vi "Post logout actions.vi"(6 "Cluster out":T2, 7 "Label.Text":string, 8 "error in (no error)":errorcluster, 9 "Caller Enqueuer":refnum<class "Message Enqueuer.lvclass">, 10 "Self Enqueuer":refnum<class "Message Enqueuer.lvclass">, 11 "ControlsIndicators":T3) -> (0 "error out":errorcluster, 3 "Cluster out":T2)   [LabVIEW 2019, in "ZenGage v3.0 UI.lvclass"]
uses:
  ZenGage v3.0 UI.lvclass
  User Interface Messages/User Interface messages/Call function_UI Msg/ButtonPress_UI.lvclass
  Type Definitions/General/UI States(UI button enable disable).ctl
  <vilib>/ActorFramework/Message Enqueuer/Message Enqueuer.lvclass
  Common/Controls/Acknowledgement.ctl
  Type Definitions/General/OutputDetails.ctl
  Type Definitions/General/Output choice.ctl
  Common/Controls/Pop-up Input.ctl
  <vilib>/ActorFramework/Message Enqueuer/Message Priority.ctl
  Type Definitions/Controls and Indicators/Select a part (combobox).ctl
  Type Definitions/Controls and Indicators/EDL control references.ctl
  Type Definitions/Controls and Indicators/Diagnostics control referencs.ctl
  Type Definitions/Controls and Indicators/Inspection control references.ctl
  Type Definitions/Controls and Indicators/General_Control references.ctl
  Type Definitions/Controls and Indicators/Controls and Indicators Cluster.ctl
  Type Definitions/General/Master sample references.ctl
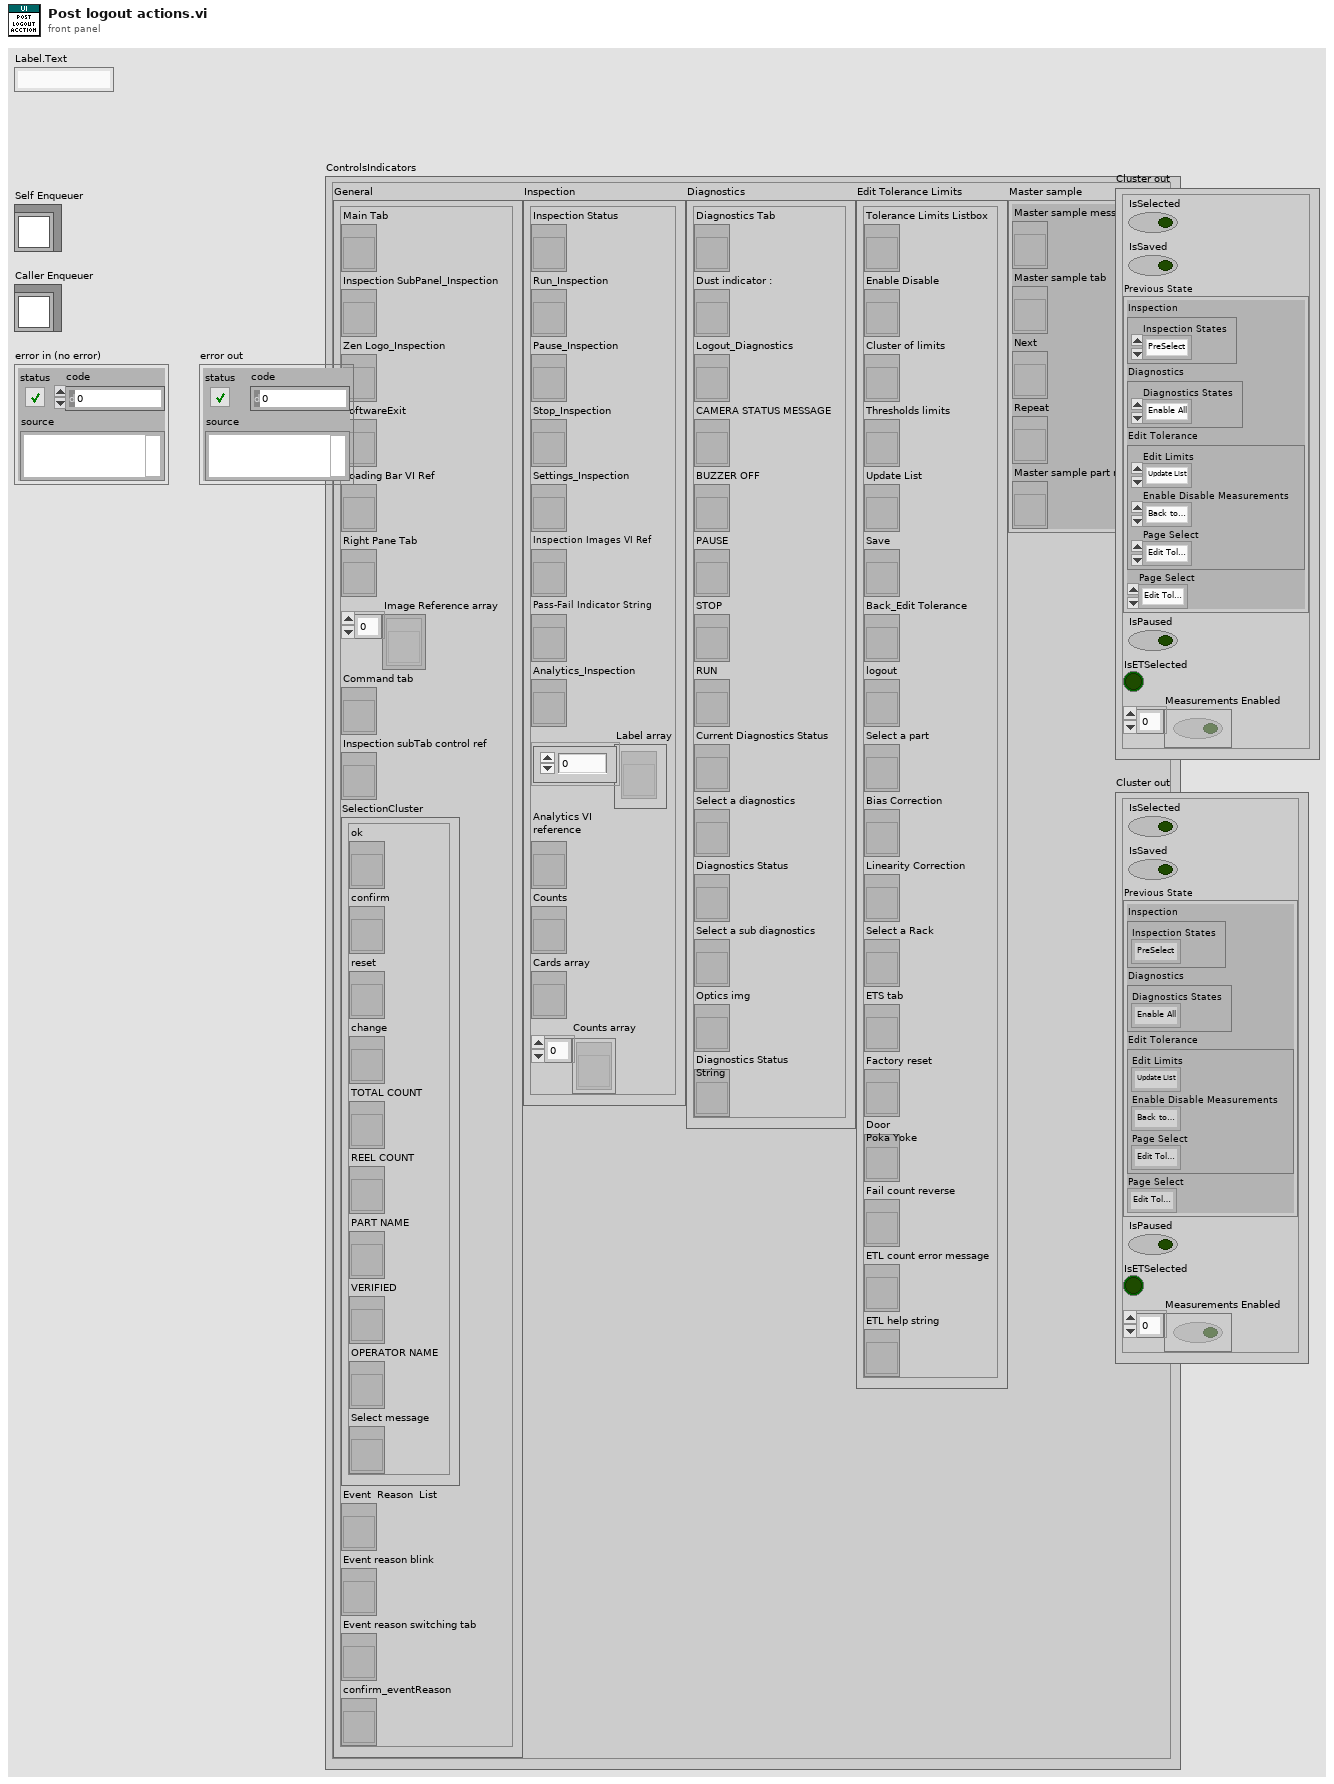
[diagram p1: front panel]
types:
  T1 = typedef "ZenGage v3.0 UI.lvclass/UI States(UI button enable disable).ctl" = cluster{"Inspection":cluster{"Inspection States":enum16{"PreSelect", "Back _Inspection", "Analytics", "Ready To Run", "Ready To Insert", "Enable All buttons", "Disable All Buttons", "Settings", "Select", "Stop", "Pause", "Inspect"}}, "Diagnostics":cluster{"Diagnostics States":enum16{"Enable All", "Camera Optics Fail", "Loading Bar", "Camera Optics", "Motor", "Arduino", "POST Done", "POST"}}, "Edit Tolerance":cluster{"Edit Limits":enum16{"Update List"}, "Enable Disable Measurements":enum16{"Back to Edit Tolerance"}, "Page Select":enum16{"Edit Tolerance Limits", "Enable Disable Buttons"}}, "Page Select":enum16{"Edit Tolerance", "Diagnostics", "Inspection"}}
  T2 = cluster{"IsSelected":bool, "IsSaved":bool, "Previous State":T1, "IsPaused":bool, "IsETSelected":bool, "Measurements Enabled":bool[]}
  T3 = typedef "ZenGage v3.0 UI.lvclass/Controls and Indicators Cluster.ctl" = cluster{"General":T4, "Inspection":T5, "Diagnostics":T6, "Edit Tolerance Limits":T7, "Master sample":T8}
  T4 = typedef "ZenGage v3.0 UI.lvclass/General_Control references.ctl" = cluster{"Main Tab":refnum<vi>, "Inspection SubPanel_Inspection":refnum<vi>, "Zen Logo_Inspection":refnum<vi>, "SoftwareExit":refnum<vi>, "Loading Bar VI Ref":refnum<vi>, "Right Pane Tab":refnum<vi>, "Image Reference array":refnum<vi>[], "Command tab":refnum<vi>, "Inspection subTab control ref":refnum<vi>, "SelectionCluster":cluster{"ok":refnum<vi>, "confirm":refnum<vi>, "reset":refnum<vi>, "change":refnum<vi>, "TOTAL COUNT":refnum<vi>, "REEL COUNT":refnum<vi>, "PART NAME":refnum<vi>, "VERIFIED":refnum<vi>, "OPERATOR NAME":refnum<vi>, "Select message":refnum<vi>}, "Event  Reason  List":refnum<vi>, "Event reason blink":refnum<vi>, "Event reason switching tab":refnum<vi>, "confirm_eventReason":refnum<vi>}
  T5 = typedef "ZenGage v3.0 UI.lvclass/Inspection control references.ctl" = cluster{"Inspection Status":refnum<vi>, "Run_Inspection":refnum<vi>, "Pause_Inspection":refnum<vi>, "Stop_Inspection":refnum<vi>, "Settings_Inspection":refnum<vi>, "Inspection Images VI Ref":refnum<vi>, "Pass-Fail Indicator String":refnum<vi>, "Analytics_Inspection":refnum<vi>, "Label array":refnum<vi>[], "Analytics VI\nreference":refnum<vi>, "Counts":refnum<vi>, "Cards array":refnum<vi>, "Counts array":refnum<vi>[]}
  T6 = typedef "ZenGage v3.0 UI.lvclass/Diagnostics control referencs.ctl" = cluster{"Diagnostics Tab":refnum<vi>, "Dust indicator :":refnum<vi>, "Logout_Diagnostics":refnum<vi>, "CAMERA STATUS MESSAGE":refnum<vi>, "BUZZER OFF":refnum<vi>, "PAUSE":refnum<vi>, "STOP":refnum<vi>, "RUN":refnum<vi>, "Current Diagnostics Status":refnum<vi>, "Select a diagnostics":refnum<vi>, "Diagnostics Status":refnum<vi>, "Select a sub diagnostics":refnum<vi>, "Optics img":refnum<vi>, "Diagnostics Status\nString":refnum<vi>}
  T7 = typedef "ZenGage v3.0 UI.lvclass/EDL control references.ctl" = cluster{"Tolerance Limits Listbox":refnum<vi>, "Enable Disable":refnum<vi>, "Cluster of limits":refnum<vi>, "Thresholds limits":refnum<vi>, "Update List":refnum<vi>, "Save":refnum<vi>, "Back_Edit Tolerance":refnum<vi>, "logout":refnum<vi>, "Select a part":refnum<vi>, "Bias Correction":refnum<vi>, "Linearity Correction":refnum<vi>, "Select a Rack":refnum<vi>, "ETS tab":refnum<vi>, "Factory reset":refnum<vi>, "Door\nPoka Yoke":refnum<vi>, "Fail count reverse":refnum<vi>, "ETL count error message":refnum<vi>, "ETL help string":refnum<vi>}
  T8 = typedef "Master sample references.ctl" = cluster{"Master sample message":refnum<vi>, "Master sample tab":refnum<vi>, "Next":refnum<vi>, "Repeat":refnum<vi>, "Master sample part message":refnum<vi>}
  T9 = enum16{"Open Logo Display", "Close Logo Display", "Open Loading Bar", "Close Loading Bar", "Open Alert Display", "Close Alert Display", "One button dialog box", "Two button dialog box", "User Authentication"}
  T10 = typedef "Pop-up Input.ctl" = cluster{"Pop-up Type":enum16{"Open Logo Display", "Close Logo Display", "Open Loading Bar", "Close Loading Bar", "Open Alert Display", "Close Alert Display", "One button dialog box", "Two button dialog box", "User Authentication"}, "Title":string, "Message":string, "Button 1 Text":string, "Button 2 Text":string, "Show Close? T/F":bool, "Title Blink? T/F":bool, "Title Blink Colour":u32}
  T11 = cluster{"Measurement\n ListBox":refnum<vi>, "Measurements Enabled":bool[]}
  T12 = enum8{"Enabled", "Disabled", "Disabled and Grayed Out"}
  T13 = typedef "ZenGage v3.0 UI.lvclass/Pop-up Output.ctl" = cluster{"Pop-up Type":enum16{"Open Logo Display", "Close Logo Display", "Open Loading Bar", "Close Loading Bar", "Open Alert Display", "Close Alert Display", "One button dialog box", "Two button dialog box", "User Authentication"}, "Message":string, "Pressed Button":string}
  T14 = typedef "ZenGage v3.0 UI.lvclass/Output choice.ctl" = enum16{"SendIgnoredFailCount", "SendPartDetails", "ButtonPress", "SendAcknowledgement", "InitiateCameraDiagnostics", "InitiateSensorDiagnostics", "SendPopupResponse", "SendEventReasonResponse", "SendErrorDetails"}
  T15 = typedef "ZenGage v3.0 UI.lvclass/OutputDetails.ctl" = cluster{"Acknowledgement_SM":T16, "Button name":string, "PartDetails":cluster{"PartName":string, "ConnectorsInReel":u64, "TotalCounts":u64, "OperatorName":string, "StampingMachineID":u32}, "SensorName":string, "CameraName":string, "PopupFeedbackDetails":cluster{"Pop-up Type":enum16{"Open Logo Display", "Close Logo Display", "Open Loading Bar", "Close Loading Bar", "Open Alert Display", "Close Alert Display", "One button dialog box", "Two button dialog box", "User Authentication"}, "Message":string, "Pressed Button":string}, "EventResponse":string, "ErrorMessage":string, "FailCountIgnore":cluster{"ReelIgnoreCount":u64, "ProductionIgnoreCount":u64}}
  T16 = typedef "Acknowledgement.ctl" = cluster{"Enqueuer":refnum<class "Message Enqueuer.lvclass">, "VIReference":refnum<vi>, "VIName":string}
  T17 = enum32{"Edit Tolerance Limits1", "Inspection", "Master sample", "Diagnostics"}
  T18 = enum32{"Analytics", "Blank", "Diagnostics", "Run", "Edit Tolerance Settings"}
  T19 = typedef "Actor Framework.lvlib/Message Enqueuer.lvclass/Message Priority.ctl" = enum16{"Low", "Normal", "High"}
  T20 = enum32{"Edit Tolerance Limits1", "Inspection", "Diagnostics"}
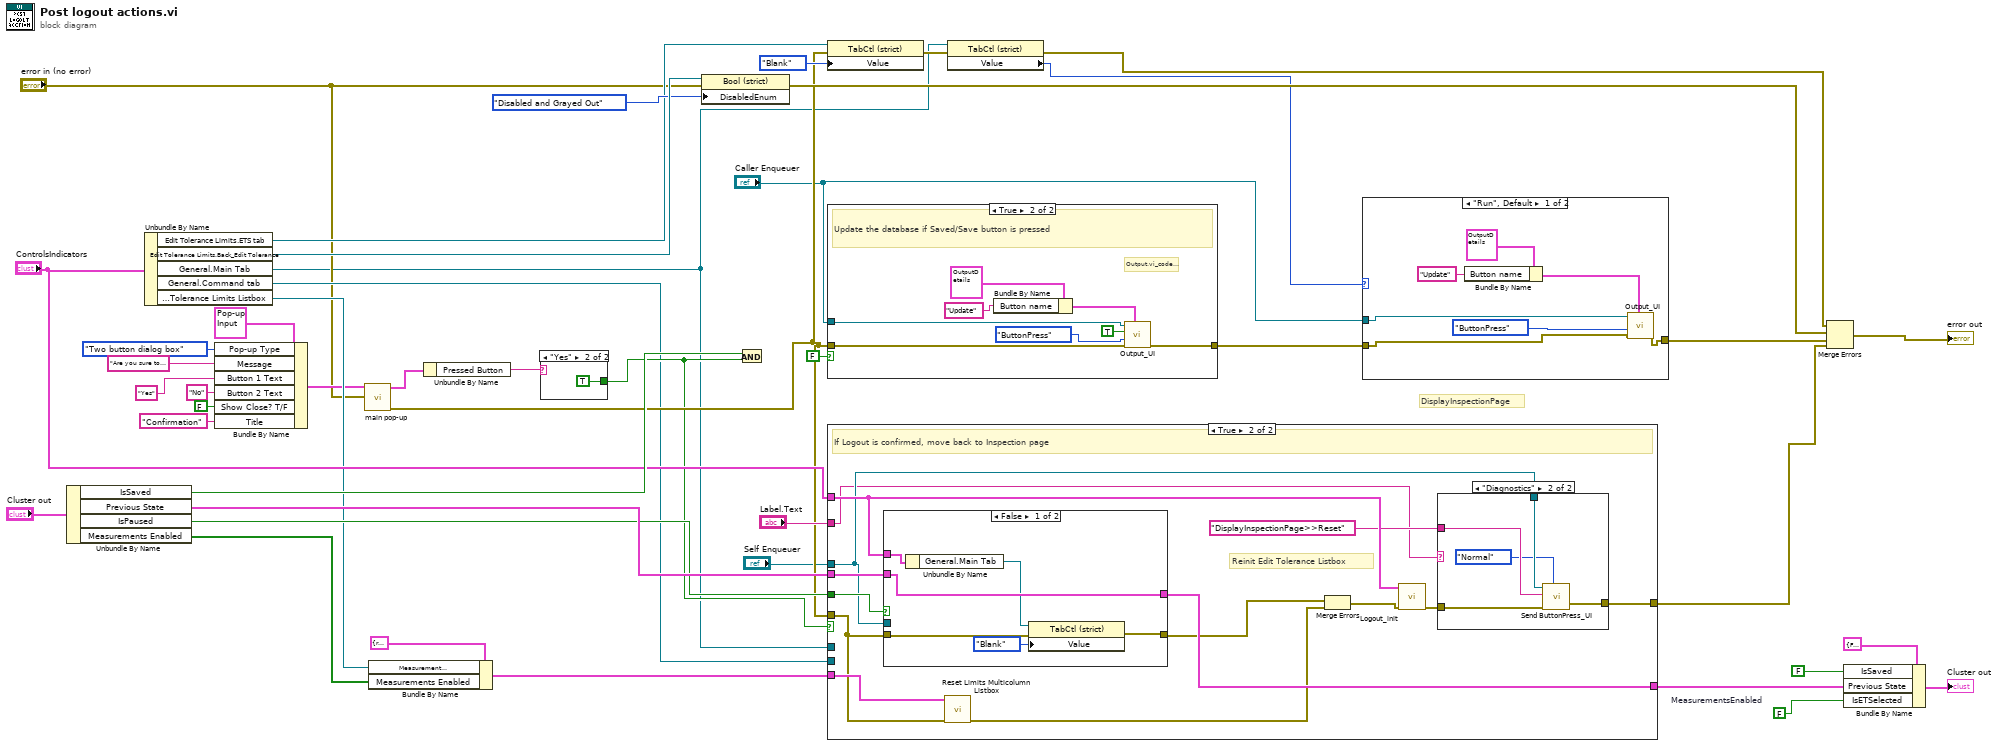
[diagram p0: block diagram]
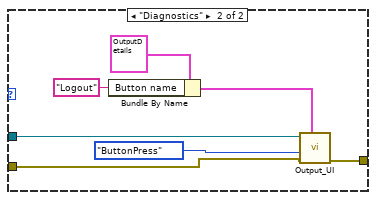
[diagram p2: hidden frame]
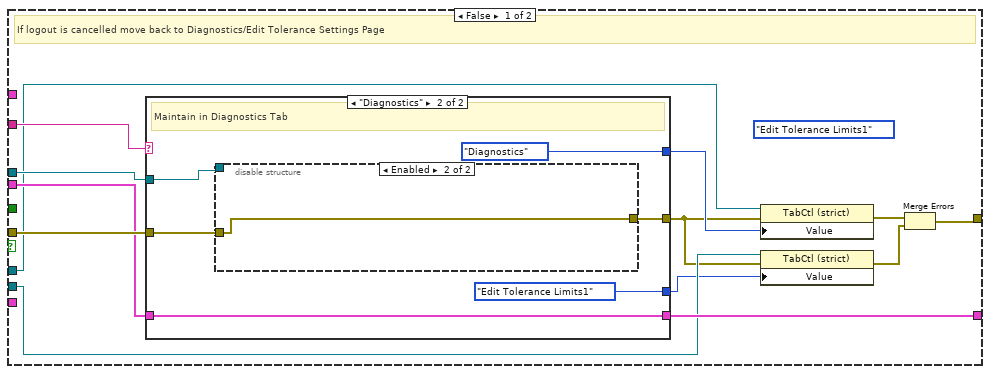
[diagram p5: hidden frame]
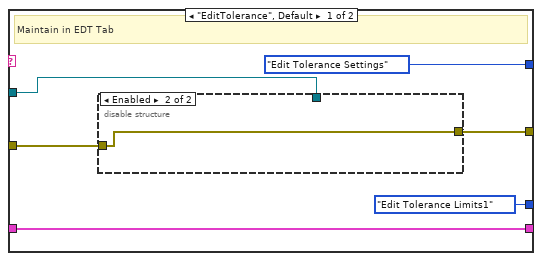
[diagram p6: hidden frame]
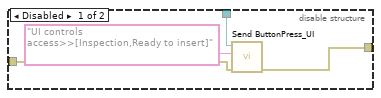
[diagram p7: hidden frame]
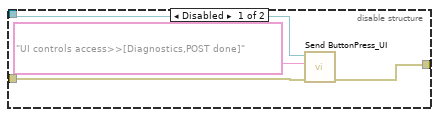
[diagram p8: hidden frame]
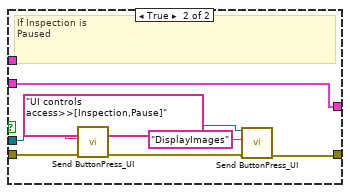
[diagram p10: hidden frame]
diagram:
  w27 = FALSE  # MeasurementsEnabled
  # "DisplayInspectionPage"
  n1 = Unbundle By Name("Cluster out") -> ("IsSaved"=w35:bool, "Previous State"=w34:T1, "IsPaused"=w33:bool, "Measurements Enabled"=w26:bool[])
  n2 = Unbundle By Name("ControlsIndicators") -> ("Edit Tolerance Limits.ETS tab"=w38:refnum<vi>, "Edit Tolerance Limits.Back_Edit Tolerance"=w41:refnum<vi>, "General.Main Tab"=w2:refnum<vi>, "General.Command tab"=w10:refnum<vi>, "Edit Tolerance Limits.Tolerance Limits Listbox"=w30:refnum<vi>)
  n3 = Bundle By Name(cluster=T10 {"Pop-up Type"=enum."Open Logo Display", "Title"="", "Message"="", "Button 1 Text"="", "Button 2 Text"="", "Show Close? T/F"=FALSE, "Title Blink? T/F"=FALSE, "Title Blink Colour"=0} ("Pop-up Input"), "Pop-up Type"=T9."Two button dialog box", "Message"="Are you sure to logout?" ("Message Input"), "Button 1 Text"="Yes" ("Boolean Text.Text"), "Button 2 Text"="No", "Show Close? T/F"=FALSE, "Title"="Confirmation") -> (w19:T10)
  n4 = call "main pop-up.vi"("error in"="error in (no error)", "Pop-up Input"=w19) -> ("error out"=w18:errorcluster, "Pop-up Output"=w17:T13)  [unwired: 8 in]
  n5 = Bundle By Name(cluster=T11 {"Measurement\n ListBox"=refnum, "Measurements Enabled"=[]} ("Cluster in"), "Measurement\n ListBox"=w30, "Measurements Enabled"=w26) -> (w25:T11)
  n6 = Unbundle By Name(w17) -> ("Pressed Button"=w16:string)
  n7 = case shown="\"Yes\"" w16 {
    tunnel: [_ TRUE] -> w15
    frame "No", Default {
    }
    frame "Yes" {
    }
  }
  n8 = property class="Bool (strict)"(reference=w41, error in="error in (no error)", "DisabledEnum"=T12."Disabled and Grayed Out" ("Disabled")) -> (error out=w39:errorcluster)  [unwired: 1 out]
  n9 = And(x=w35, y=w15) -> ()  [unwired: 1 out]
  n10 = property class="TabCtl (strict)"(reference=w38, error in=w18, "Value"=enum32{"Display", "Blank"}."Blank") -> (error out=w5:errorcluster)  [unwired: 1 out]
  n11 = case shown="True" FALSE {
    tunnel: "Caller Enqueuer" -> [_ w50]
    tunnel: w18 -> [w47 w55]
    tunnel: [w47 w54] -> w8
    frame False {
    }
    frame True {
      # "Output.vi_code modified (02-08-2018)"
      # "Update the database if Saved/Save button is pressed"
      n12 = Bundle By Name(cluster=T15 {"Acknowledgement_SM"={"Enqueuer"=refnum, "VIReference"=refnum, "VIName"=""}, "Button name"="", "PartDetails"={"PartName"="", "ConnectorsInReel"=0, "TotalCounts"=0, "OperatorName"="", "StampingMachineID"=0}, "SensorName"="", "CameraName"="", "PopupFeedbackDetails"={"Pop-up Type"=enum."Open Logo Display", "Message"="", "Pressed Button"=""}, "EventResponse"="", "ErrorMessage"="", "FailCountIgnore"={"ReelIgnoreCount"=0, "ProductionIgnoreCount"=0}} ("OutputDetails"), "Button name"="Update") -> (w51:T15)
      n13 = call "Output_UI.vi"("OutputDetails"=w51, "error in"=w55, "Functionality"=Output_choice."ButtonPress", "Testbench"=TRUE, "SMEnqueuer"=w50) -> ("error out"=w54:errorcluster)  [unwired: 6 in]
    }
  }
  n14 = case shown="True" w15 {
    tunnel: [w57 w94] -> w11
    tunnel: w18 -> [w67 w102]
    tunnel: "Label.Text" -> [w68 w91]
    tunnel: [w66 w99] -> w45
    tunnel: w34 -> [w65 w100]
    tunnel: w33 -> [_ w104]
    tunnel: "Self Enqueuer" -> [w64 w93]
    tunnel: "ControlsIndicators" -> [_ w101]
    tunnel: w25 -> [_ w103]
    tunnel: w2 -> [w63 _]
    tunnel: w10 -> [w61 _]
    frame False {
      (unwired) T20."Edit Tolerance Limits1" ("Value")
      # "If logout is cancelled move back to Diagnostics/Edit Tolerance Settings Page"
      n15 = case shown="\"Diagnostics\"" w68 {
        tunnel: w67 -> [w72 w84]
        tunnel: [w71 w83] -> w60
        tunnel: [w73 w82] -> w66
        tunnel: [T18."Edit Tolerance Settings" ("Value") T18."Diagnostics" ("Value")] -> w62
        tunnel: w65 -> [w73 w82]
        tunnel: w64 -> [w70 w81]
        tunnel: [T17."Edit Tolerance Limits1" ("Value") T17."Edit Tolerance Limits1" ("Value")] -> w56
        frame "EditTolerance", Default {
          # "Maintain in EDT Tab"
          n16 = disable-structure shown="Enabled" {
            disable-tunnel: w72 -> [w78 w79]
            disable-tunnel: [w77 w79] -> w71
            disable-tunnel: w70 -> [w76 _]
            frame Disabled {
              n17 = call "Send ButtonPress_UI.vi"("error in (no error)"=w78, "FunctionalityName"="UI controls access>>[Inspection,Ready to insert]" ("Functionality name"), "Message Enqueuer"=w76) -> ("error out"=w77:errorcluster)  [unwired: 7 in, 1 out]
            }
            frame Enabled {
            }
          }
        }
        frame "Diagnostics" {
          # "Maintain in Diagnostics Tab"
          n18 = disable-structure shown="Enabled" {
            disable-tunnel: w84 -> [w89 w90]
            disable-tunnel: [w88 w90] -> w83
            disable-tunnel: w81 -> [w87 _]
            frame Disabled {
              n19 = call "Send ButtonPress_UI.vi"("error in (no error)"=w89, "FunctionalityName"="UI controls access>>[Diagnostics,POST done]" ("Functionality name"), "Message Enqueuer"=w87) -> ("error out"=w88:errorcluster)  [unwired: 7 in, 1 out]
            }
            frame Enabled {
            }
          }
        }
      }
      n20 = property class="TabCtl (strict)"(reference=w63, error in=w60, "Value"=w62) -> (error out=w59:errorcluster)  [unwired: 1 out]
      n21 = property class="TabCtl (strict)"(reference=w61, error in=w60, "Value"=w56) -> (error out=w58:errorcluster)  [unwired: 1 out]
      n22 = Merge Errors(w59, w58) -> (w57:errorcluster)
    }
    frame True {
      # "Reinit Edit Tolerance Listbox"
      # "If Logout is confirmed, move back to Inspection page"
      n23 = case shown="False" w104 {
        tunnel: [w116 w124] -> w99
        tunnel: w100 -> [w116 w124]
        tunnel: w102 -> [w114 w122]
        tunnel: [w113 w118] -> w97
        tunnel: w93 -> [_ w121]
        tunnel: w101 -> [w115 _]
        frame False {
          n24 = Unbundle By Name(w115) -> ("General.Main Tab"=w112:refnum<vi>)
          n25 = property class="TabCtl (strict)"(reference=w112, error in=w114, "Value"=T18."Blank") -> (error out=w113:errorcluster)  [unwired: 1 out]
        }
        frame True {
          # "If Inspection is\nPaused"
          n26 = call "Send ButtonPress_UI.vi"("error in (no error)"=w122, "FunctionalityName"="UI controls access>>[Inspection,Pause]", "Message Enqueuer"=w121) -> ("error out"=w119:errorcluster, "Message Enqueuer out"=w117:refnum<class "Message Enqueuer.lvclass">)  [unwired: 7 in]
          n27 = call "Send ButtonPress_UI.vi"("error in (no error)"=w119, "FunctionalityName"="DisplayImages", "Message Enqueuer"=w117) -> ("error out"=w118:errorcluster)  [unwired: 7 in, 1 out]
        }
      }
      n28 = call "Reset Limits Multicolumn Listbox.vi"("error in (no error)"=w102, "Cluster in"=w103) -> ("error out"=w98:errorcluster)  [unwired: 9 in]
      n29 = Merge Errors(w97, w98) -> (w96:errorcluster)
      n30 = call "Logout_init.vi"("error in (no error)"=w96, "ZenGage v3.0 UI in"=w101) -> ("error out"=w95:errorcluster)  [unwired: 9 in]
      n31 = case shown="\"Diagnostics\"" w91 {
        tunnel: w95 -> [w105 w110]
        tunnel: [w105 w109] -> w94
        tunnel: w93 -> [_ w108]
        tunnel: "DisplayInspectionPage>>Reset" ("Button name") -> [_ w107]
        frame "EditTolerance", Default {
        }
        frame "Diagnostics" {
          n32 = call "Send ButtonPress_UI.vi"("Message Priority (Normal)"=Message_Priority."Normal", "error in (no error)"=w110, "FunctionalityName"=w107, "Message Enqueuer"=w108) -> ("error out"=w109:errorcluster)  [unwired: 6 in, 1 out]
        }
      }
    }
  }
  n33 = property class="TabCtl (strict)"(reference=w2, error in=w5) -> (error out=w4:errorcluster, "Value"=w3:T18)  [unwired: 1 out]
  n34 = case shown="\"Run\", Default" w3 {
    tunnel: w8 -> [w126 w138]
    tunnel: [w127 w137] -> w7
    tunnel: "Caller Enqueuer" -> [w125 w136]
    frame "Run", Default {
      n35 = Bundle By Name(cluster=T15 {"Acknowledgement_SM"={"Enqueuer"=refnum, "VIReference"=refnum, "VIName"=""}, "Button name"="", "PartDetails"={"PartName"="", "ConnectorsInReel"=0, "TotalCounts"=0, "OperatorName"="", "StampingMachineID"=0}, "SensorName"="", "CameraName"="", "PopupFeedbackDetails"={"Pop-up Type"=enum."Open Logo Display", "Message"="", "Pressed Button"=""}, "EventResponse"="", "ErrorMessage"="", "FailCountIgnore"={"ReelIgnoreCount"=0, "ProductionIgnoreCount"=0}} ("OutputDetails"), "Button name"="Update") -> (w128:T15)
      n36 = call "Output_UI.vi"("OutputDetails"=w128, "error in"=w126, "Functionality"=Output_choice."ButtonPress", "SMEnqueuer"=w125) -> ("error out"=w127:errorcluster)  [unwired: 7 in]
    }
    frame "Diagnostics" {
      n37 = Bundle By Name(cluster=T15 {"Acknowledgement_SM"={"Enqueuer"=refnum, "VIReference"=refnum, "VIName"=""}, "Button name"="", "PartDetails"={"PartName"="", "ConnectorsInReel"=0, "TotalCounts"=0, "OperatorName"="", "StampingMachineID"=0}, "SensorName"="", "CameraName"="", "PopupFeedbackDetails"={"Pop-up Type"=enum."Open Logo Display", "Message"="", "Pressed Button"=""}, "EventResponse"="", "ErrorMessage"="", "FailCountIgnore"={"ReelIgnoreCount"=0, "ProductionIgnoreCount"=0}} ("OutputDetails"), "Button name"="Logout") -> (w132:T15)
      n38 = call "Output_UI.vi"("OutputDetails"=w132, "error in"=w138, "Functionality"=Output_choice."ButtonPress", "SMEnqueuer"=w136) -> ("error out"=w137:errorcluster)  [unwired: 7 in]
    }
  }
  n39 = Merge Errors(w4, w39, w7, w11) -> (→"error out":errorcluster)
  n40 = Bundle By Name(cluster=T2 {"IsSelected"=FALSE, "IsSaved"=FALSE, "Previous State"={"Inspection"={"Inspection States"=enum."PreSelect"}, "Diagnostics"={"Diagnostics States"=enum."Enable All"}, "Edit Tolerance"={"Edit Limits"=enum."Update List", "Enable Disable Measurements"=enum."Back to Edit Tolerance", "Page Select"=enum."Edit Tolerance Limits"}, "Page Select"=enum."Edit Tolerance"}, "IsPaused"=FALSE, "IsETSelected"=FALSE, "Measurements Enabled"=[]} ("Cluster out"), "IsSaved"=FALSE ("Edit Tolerance Settings Cluster.Saved?"), "Previous State"=w45, "IsETSelected"=w27) -> (→"Cluster out":T2)
